vi "class_data.vi"() -> ()   [LabVIEW 2010, in "GenericStage.lvclass"]
uses:
  GenericStage.lvclass
panel:
  in  "latest instance":refnum<class "GenericStage.lvclass">
  in  "translation request queue name":string="translation request queue"
  in  "locked by":string
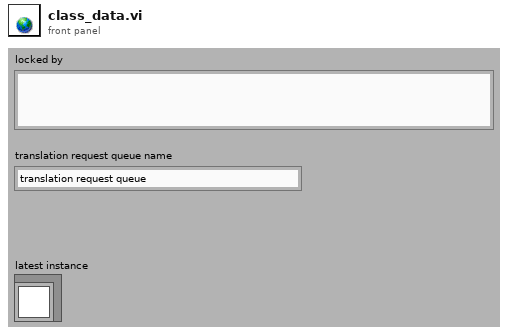
[diagram p1: front panel]
diagram:
